vi "float2str.vi"(10 "precision":ext, 11 "float":ext) -> (3 "string":string)   [LabVIEW 2017]
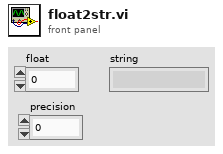
[diagram p1: front panel]
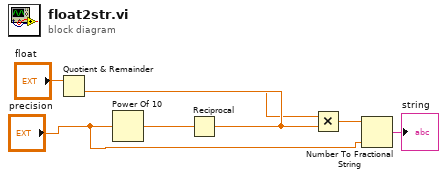
[diagram p0: block diagram]
diagram:
  n1 = Power Of 10(x="precision") -> (10^x=w3:ext)
  n2 = Reciprocal(x=w3) -> (1/x=w4:ext)
  n3 = Quotient & Remainder(x="float", y=w4) -> (floor(x/y)=w2:ext)  [unwired: 1 out]
  n4 = Multiply(x=w2, y=w4) -> (x*y=w7:ext)
  n5 = Number To Fractional String(number=w7, precision (6)="precision") -> (F-format string=→"string":string)  [unwired: 2 in]
